vi "DB Tools Select Data (fast Quarry).vi"(6 "optional clause":string, 7 "Use Fast quarry":bool, 8 "error in (no error)":errorcluster, 9 "columns":string[](array[string]), 10 "table":string, 11 "connection reference":T1) -> (0 "error out":errorcluster, 1 "data":variant[][](array[variant]), 2 "Data out":string[][](table), 3 "connection reference out":T1)   [LabVIEW 2009]
doc: "Selects data from the <B>table</B> in the database identified by <B>connection reference</B> using the columns supplied in the <B>columns</B> array."
uses:
  <vilib>/addons/database/Connection.llb/Conn ObjectReference.ctl
  <vilib>/addons/database/Recordset.llb/Rec Destroy - Connection.vi
  <vilib>/addons/database/Recordset.llb/Rec Fetch Recordset Data (R).vi
  <vilib>/addons/database/Connection.llb/Conn Execute.vi
  <vilib>/addons/database/NI_Database_API.lvlib
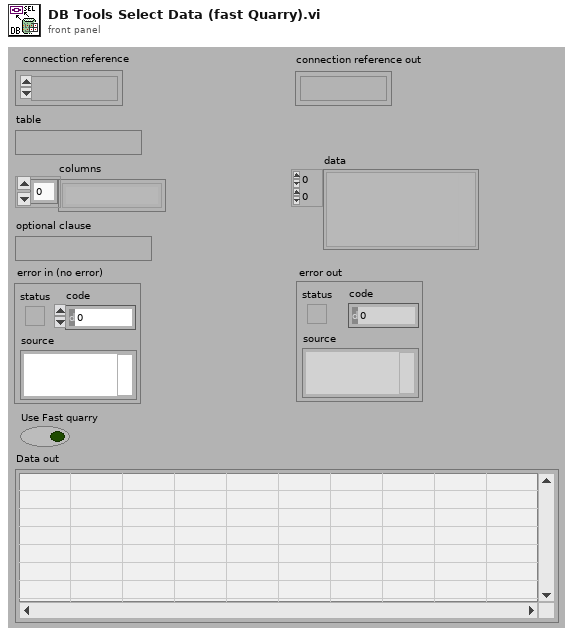
[diagram p1: front panel]
types:
  T1 = typedef "NI_Database_API.lvlib/Conn ObjectReference.ctl" = refnum<k1>
  T2 = typedef "NI_Database_API.lvlib/Rec ObjectReference.ctl" = refnum<k1>
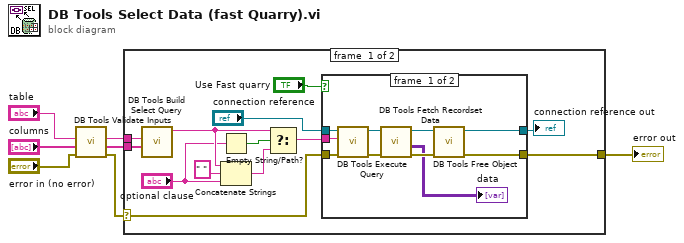
[diagram p0: block diagram]
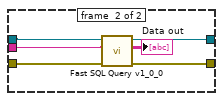
[diagram p2: hidden frame]
diagram:
  n1 = call <vilib>:"DB Tools Validate Inputs.vi"("error in (no error)"="error in (no error)", "columns"="columns", "table"="table") -> ("error out"=w2:errorcluster, "columns out"=w4:string[], "table out"=w3:string)  [unwired: 2 in]
  n2 = case shown="No Error" w2 {
    selector: w2 -> [w18 w37]
    tunnel: w4 -> [w20 _]
    tunnel: w3 -> [w19 _]
    tunnel: [w17 w37] -> w5
    frame #0 {
      n3 = call <vilib>:"DB Tools Build Select Query.vi"("columns"=w20, "table name"=w19) -> ("select query"=w14:string)  [unwired: 5 in]
      n4 = Empty String/Path?(string/path="optional clause") -> (empty?=w15:bool)
      n5 = Concatenate Strings(w14, " " ("Substring"), "optional clause") -> (w13:string)
      n6 = Select(t=w14, s=w15, f=w13) -> (s? t:f=w10:string)
      n7 = case shown="True" "Use Fast quarry" {
        tunnel: w18 -> [w30 w34]
        tunnel: [w29 w35] -> w17
        tunnel: "connection reference" -> [w23 w33]
        tunnel: w10 -> [w22 w32]
        tunnel: [w21 w36] -> w8
        frame #0 {
          n8 = call-poly <vilib>:"DB Tools Execute Query.vi"("error in (no error)"=w30, "SQL query"=w22, "connection reference"=w23) -> ("error out"=w26:errorcluster, "recordset reference"=w27:T2)  [unwired: 5 in]
          n9 = call-poly <vilib>:"DB Tools Fetch Recordset Data.vi"("error in (no error)"=w26, "recordset reference"=w27) -> ("error out"=w25:errorcluster, "recordset data"=→"data":variant[][], "recordset reference out"=w28:T2)  [unwired: 3 in]
          n10 = call-poly <vilib>:"DB Tools Free Object.vi"("error in (no error)"=w25, "recordset reference"=w28) -> ("error out"=w29:errorcluster, "connection reference"=w21:T1)  [unwired: 8 in]
        }
        frame #1 {
          n11 = call "Fast SQL Query v1_0_0.vi"("error in (no error)"=w34, "SQL"=w32, "connection reference"=w33) -> ("error out"=w35:errorcluster, "2D Data out"=→"Data out":string[][], "dup connection reference"=w36:T1)  [unwired: 4 in, 2 out]
        }
      }
      "connection reference out" <- w8
    }
    frame #1 {
    }
  }
  "error out" <- w5
